vi "Configure Clock_5160.vi"(8 "error in":errorcluster, 10 "Clock Source":T1(ring), 11 "FPGA VI Reference in":T2) -> (0 "error out":errorcluster, 2 "Configuration Error":bool, 3 "FPGA VI Reference Out":T2)   [LabVIEW 2013]
doc: "This VI configures the clock source for the NI 5772. For execution steps, refer to the comments on the block diagram."
uses:
  5160FPGAref.ctl
  <vilib>/rvi/interface/common/niFpgaWaitOnOcc.vi
  <vilib>/Utility/error.llb/Error Cluster From Error Code.vi
  <vilib>/rvi/errors/niLvFpgaAdjustHostInterfaceError.vi
  <vilib>/rvi/interface/nirviReadWriteControl/nirviReadWriteControl.xnode
  NiFpgaLv.dll
  <vilib>/rvi/interface/Simulation/niFpgaSimulationCallBeginRW.vi
panel:
  # "This VI configures the clock source for the NI 5771. For execution steps, refer to the comments on the block diagram."
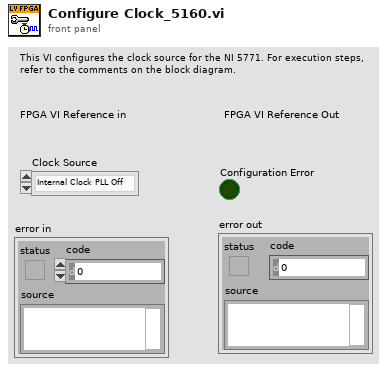
[diagram p1: front panel]
types:
  T1 = enum8{"Internal Clock PLL Off", "Internal Clock PLL On (REF IN)", "External Clock (CLK_IN)", "Internal Clock PLL On (IoModSyncClk)"}
  T2 = typedef "5160FPGAref.ctl" = refnum<k20>
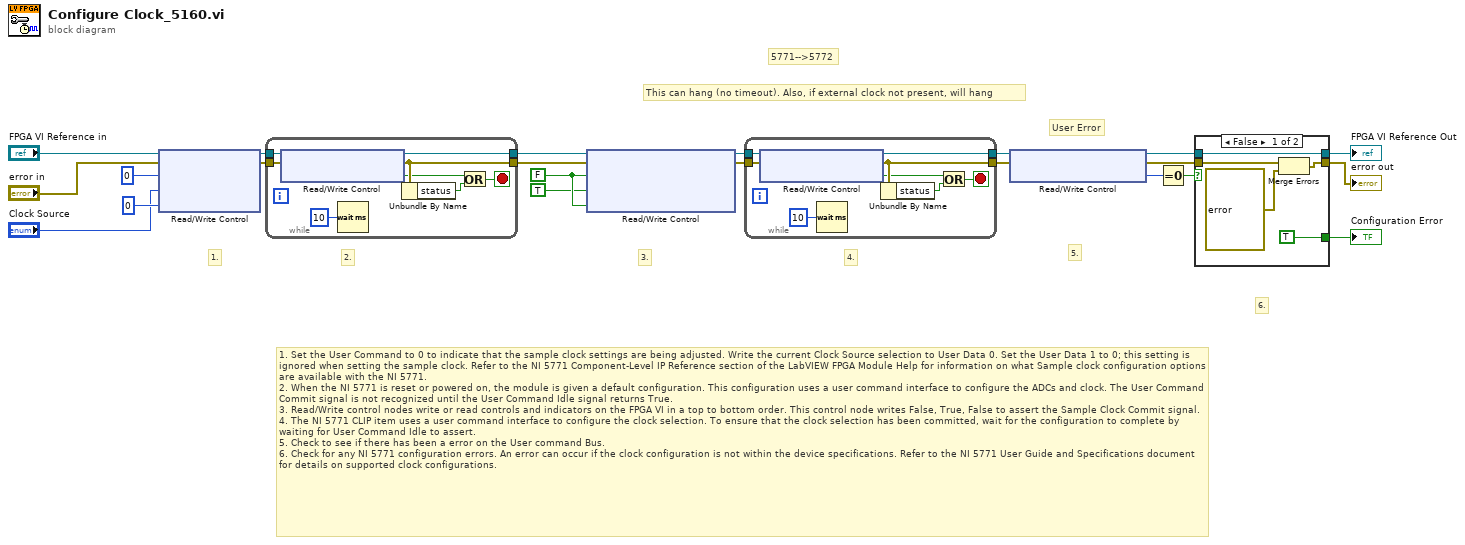
[diagram p0: block diagram]
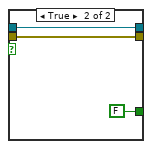
[diagram p2: hidden frame]
diagram:
  w17 = FALSE ("Sample Clock Commit")
  # "User Error"
  # "5771-->5772"
  # "This can hang (no timeout). Also, if external clock not present, will hang"
  # "6."
  # "1. Set the User Command to 0 to indicate that the sample clock settings are being adjusted. Write the current Clock Source selection to User Data 0. Set the User Data 1 to 0; this setting is ignored when setting the sample clock. Refer to the NI 5771 Component-Level IP Reference section of the LabVIEW FPGA Module Help for information on what Sample clock configuration options are available with the NI 5771.\n2. When the NI 5771 is reset or powered on, the module is given a default configuration. This configuration uses a user command interface to configure the ADCs and clock. The User Command Commit signal is not recognized until the User Command Idle signal returns True.\n3. Read/Write control nodes write or read controls and indicators on the FPGA VI in a top to bottom order. This control node writes False, True, False to assert the Sample Clock Commit signal.\n4. The NI 5771 CLIP item uses a user command interface to configure the clock selection. To ensure that the clock selection has been committed, wait for the configuration to complete by waiting for User Command Idle to assert.\n5. Check to see if there has been a error on the User command Bus. \n6. Check for any NI 5771 configuration errors. An error can occur if the clock configuration is not within the device specifications. Refer to the NI 5771 User Guide and Specifications document for details on supported clock configurations."
  # "5."
  # "4."
  # "3."
  # "2."
  # "1."
  n1 = xnode "Read/Write Control"("FPGA VI Reference In"="FPGA VI Reference in", "error in"="error in", "User Command"=u8 0, "User Data 0"="Clock Source", "User Data 1"=u8 0) -> ("FPGA VI Reference Out"=w21:T2, "error out"=w20:errorcluster)
  n2 = while {
    tunnel: w21 -> [w26]
    tunnel: w20 -> [w27]
    tunnel: [w24] -> w18
    tunnel: [w25] -> w19
    stop <- w28 stop-if-true
    n3 = xnode "Read/Write Control"("FPGA VI Reference In"=w26, "error in"=w27) -> ("FPGA VI Reference Out"=w25:T2, "error out"=w24:errorcluster, "User Command Idle"=w23:bool)
    n4 = Wait (ms)(milliseconds to wait=u32 10) -> ()  [unwired: 1 out]
    n5 = Unbundle By Name(w24) -> ("status"=w29:bool)
    n6 = Or(x=w23, y=w29) -> (x .or. y?=w28:bool)
  }
  n7 = xnode "Read/Write Control"("FPGA VI Reference In"=w19, "error in"=w18, "User Command Commit"=w17, "User Command Commit"=TRUE ("Sample Clock Commit"), "User Command Commit"=w17) -> ("FPGA VI Reference Out"=w14:T2, "error out"=w13:errorcluster)
  n8 = while {
    tunnel: w14 -> [w34]
    tunnel: w13 -> [w35]
    tunnel: [w32] -> w12
    tunnel: [w33] -> w11
    stop <- w36 stop-if-true
    n9 = xnode "Read/Write Control"("FPGA VI Reference In"=w34, "error in"=w35) -> ("FPGA VI Reference Out"=w33:T2, "error out"=w32:errorcluster, "User Command Idle"=w31:bool)
    n10 = Wait (ms)(milliseconds to wait=u32 10) -> ()  [unwired: 1 out]
    n11 = Unbundle By Name(w32) -> ("status"=w37:bool)
    n12 = Or(x=w31, y=w37) -> (x .or. y?=w36:bool)
  }
  n13 = xnode "Read/Write Control"("FPGA VI Reference In"=w11, "error in"=w12) -> ("FPGA VI Reference Out"=w4:T2, "error out"=w8:errorcluster, "User Command Status"=w7:u8)
  n14 = Equal To 0?(x=w7) -> (x = 0?=w6:bool)
  n15 = case shown="False" w6 {
    tunnel: [w43 w46] -> w2
    tunnel: w8 -> [w42 w46]
    tunnel: [TRUE ("Configured?") FALSE ("Configured?")] -> w1
    tunnel: w4 -> [w39 w44]
    tunnel: [w39 w44] -> w3
    frame False {
      n16 = Merge Errors(w42, errorcluster {"status"=TRUE, "code"=-8998, "source"="IO Module clock not configured correctly. Please ensure that the desired clock meets the required specifications."} ("error in")) -> (w43:errorcluster)
    }
    frame True {
    }
  }
  "error out" <- w2
  "FPGA VI Reference Out" <- w3
  "Configuration Error" <- w1
